vi "DataArrayTest.vi"() -> ()   [LabVIEW 2024]
uses:
  <vilib>/Utility/file.llb/Write Delimited Spreadsheet (string).vi
panel:
  out "appended array 2":string[][](array[string])
  out "output array":string[](array[string])
  out "Array 2":string[](array[string])
  in  "stop":bool
  out "appended array":dbl[][](array[numeric])
  out "Array":dbl[](array[numeric])
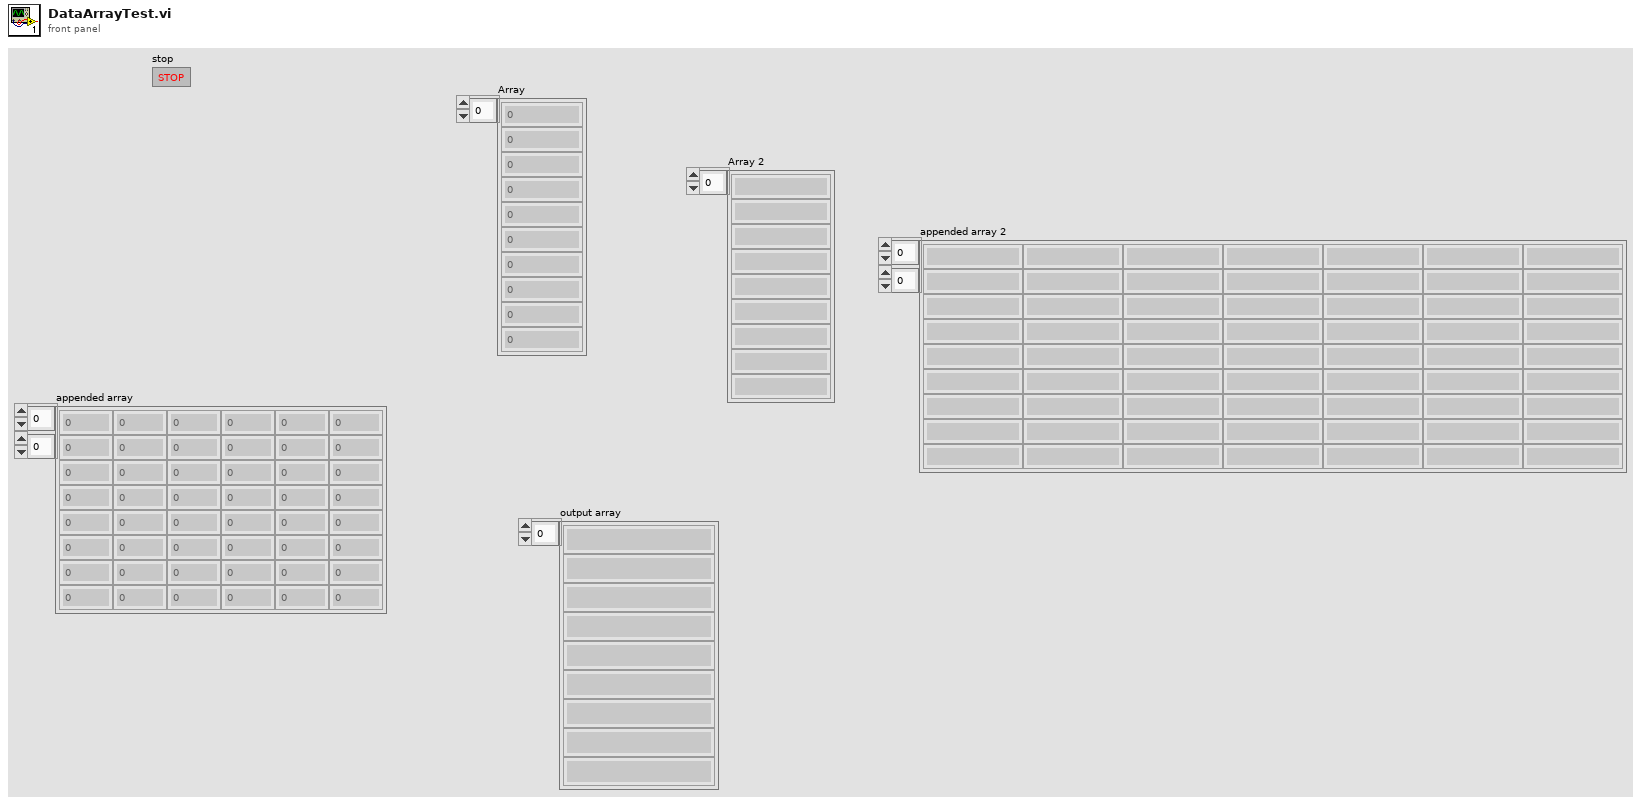
[diagram p1: front panel]
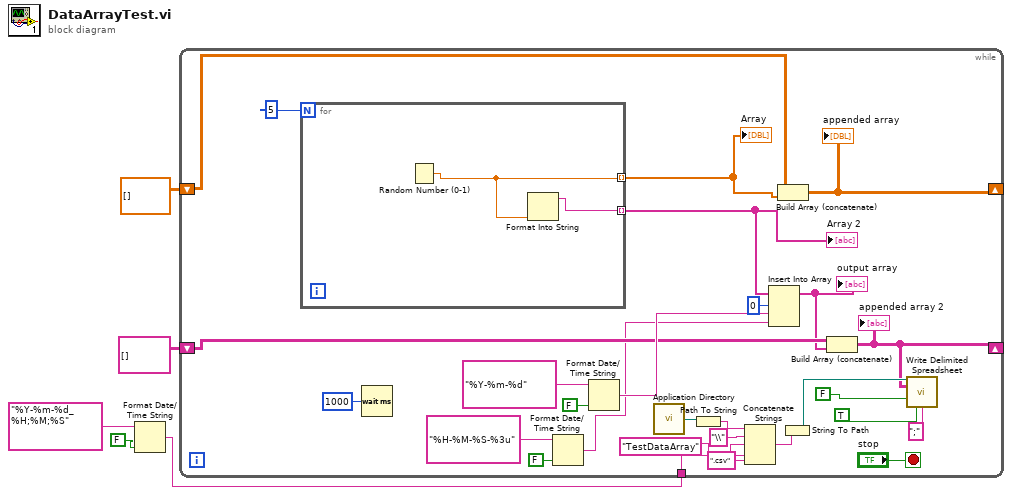
[diagram p0: block diagram]
diagram:
  n1 = Format Date/Time String(time format string (%c)="%Y-%m-%d_%H;%M;%S", UTC format=FALSE) -> (date/time string=w1:string)  [unwired: 1 in]
  n2 = while {
    shift-right: [w30] -> _
    shift-left: dbl[][] [] -> [w29]
    shift-right: [w13] -> _
    shift-left: string[][] [] -> [w23]
    tunnel: w1 -> [w7]
    stop <- "stop" stop-if-true
    n3 = for {
      N: 5 -> [_]
      tunnel: [w35] -> w31 mode=indexing
      tunnel: [w34] -> w26 mode=indexing
      n4 = Random Number (0-1)() -> (number: 0 to 1=w35:dbl)
      n5 = Format Into String(w35) -> (resulting string=w34:string)  [unwired: 3 in, 1 out]
    }
    "Array" <- w31
    "Array 2" <- w26
    n6 = Wait (ms)(milliseconds to wait=u32 1000) -> ()  [unwired: 1 out]
    n7 = Format Date/Time String(time format string (%c)="%H-%M-%S-%3u", UTC format=FALSE) -> (date/time string=w10:string)  [unwired: 1 in]
    n8 = Format Date/Time String(time format string (%c)="%Y-%m-%d", UTC format=FALSE) -> (date/time string=w24:string)  [unwired: 1 in]
    n9 = call <vilib>:"Application Directory.vi"() -> ("Application Directory"=w21:path)
    n10 = Path To String(path=w21) -> (string=w20:string)
    n11 = Concatenate Strings(w20, "\\" ("string"), "TestDataArray" ("string"), w7, ".csv" ("string")) -> (w19:string)
    n12 = Insert Into Array(array=w26, index=0, new element #1=w24, new element #2=w10) -> (w15:string[])
    "output array" <- w15
    n13 = Build Array (concatenate)(w29, w31) -> (w30:dbl[][])
    "appended array" <- w30
    n14 = String To Path(string=w19) -> (path=w18:path)
    n15 = Build Array (concatenate)(w23, w15) -> (w13:string[][])
    "appended array 2" <- w13
    n16 = call-poly <vilib>:"Write Delimited Spreadsheet.vi"("file path (dialog if empty)"=w18, "2D data"=w13, "append to file? (new file:F)"=FALSE, "transpose? (no:F)"=TRUE, "delimiter (\\t)"=";" ("delimiter (\\t)")) -> ()  [unwired: 9 in, 2 out]
  }
